vi "Median Filter.vi"(0 "Values":dbl[](array[numeric])=[5737.7244576537305, 5716.134924134484, 5694.815267577043, 5673.76167217572, 5652.9704006512275, 5632.437792319555, 5612.160261218363, 5592.1342942889905, 5572.356449612099, 5552.823354695204, 5533.531704810249, 5514.478261379612, 5495.659850408876, 5477.073360964807, 5458.7157436970465, 5440.584009402092, 5422.675227628114, 5404.98652531934, 5387.515085498669, 5370.258145987328, 5353.212998160276, 5336.376985736356, 5319.747503601926, 5303.3219966670285, 5287.097958752993, 5271.072931510506, 5255.2445033672175, 5239.610308503905, 5224.168025858348, 5208.915378156069, 5193.850130967058, 5178.970091787739, 5164.273109147386, 5149.757071738242, 5135.419907568635, 5121.259583138374, 5107.274102635845, 5093.461507155978, 5079.819873938706, 5066.347315627092, 5053.041979544701, 5039.902046991551, 5026.92573255817, 5014.111283457203, 5001.4569788720555, 4988.9611293221105, 4976.622076044022, 4964.438190388647, 4952.407873233138, 4940.529554407835, 4928.801692137438, 4917.222772496194, 50001.0, 50001.0, 50001.0, 50001.0, 50001.0, 50001.0, 50001.0, 50001.0, 50001.0, 50001.0, 50001.0, 50001.0, 50001.0, 50001.0, 50001.0, 50001.0, 50001.0, 50001.0, 50001.0, 50001.0, 50001.0, 50001.0, 50001.0, 50001.0, 50001.0, 50001.0, 50001.0, 50001.0, 50001.0, 50001.0, 50001.0, 50001.0, 50001.0, 50001.0, 50001.0, 50001.0, 50001.0, 50001.0, 50001.0, 50001.0, 50001.0, 50001.0, 50001.0, 50001.0, 50001.0, 50001.0, 50001.0, 50001.0, 50001.0, 50001.0, 50001.0, 50001.0, 50001.0, 50001.0, 50001.0, 50001.0, 50001.0, 50001.0, 50001.0, 50001.0, 50001.0, 50001.0, 50001.0, 50001.0, 50001.0, 50001.0, 50001.0, 50001.0, 50001.0, 50001.0, 50001.0, 50001.0, 50001.0, 50001.0, 50001.0, 50001.0, 50001.0, 50001.0, 50001.0, 50001.0, 50001.0, 50001.0, 50001.0, 50001.0, 50001.0, 50001.0, 50001.0, 50001.0, 50001.0, 50001.0, 50001.0, 50001.0, 4138.36385992044, 4148.764027757794, 4159.2959873554555, 4169.961147536824, 4180.760943269987, 4191.6968361984045, 4202.7703151853475, 4213.982896872684, 4225.336126254318, 4236.831577264759, 4248.470853383298, 4260.255588254225, 4272.187446323593, 4284.268123493028, 4296.499347791133, 4308.88288006296, 4321.420514678189, 4334.114080258547, 4346.965440425061, 4359.976494565826, 4373.149178624846, 4386.485465912698, 4399.987367939662, 4413.656935272053, 4427.496258412496, 4441.507468704933, 4455.69273926514, 4470.054285937593, 4484.594368279553, 4499.315290573274, 4514.219402867235, 4529.309102047392, 4544.586832939442, 4560.055089443108, 4575.716415699603, 4591.573407293312, 4607.628712488913, 4623.885033505139, 4640.345127826415, 4657.011809553725, 4673.887950796052, 4690.976483103799, 4708.280398945661, 4725.802753230531, 4743.546664875976, 4761.515318424989, 4779.711965712726, 4798.139927585015, 4816.802595670585, 4835.703434208887, 4854.845981935558, 4874.233854027718, 4893.870744111253, 4913.760426332378, 4933.906757495931, 4954.3136792729265, 4974.985220479884, 4995.925499432786, 5017.13872637844, 5038.629206006256, 5060.401340043521, 5082.459629937463, 5104.808679627467, 5127.45319841095, 5150.398003906725, 5173.648025119562, 5197.208305610149, 5221.084006774594, 5245.280411237951, 5269.802926366389, 5294.657087902874, 5319.8485637314425, 5345.3831577754045, 5371.266814035074, 5397.505620770815, 5424.105814837618, 5451.0737861775815, 5478.416082477071, 5506.13941399559, 5534.250658573846, 5549.557682605477, 5530.795421099543, 5512.264189130301, 5493.960970097327, 5475.882806682313, 5458.026799481461, 5440.39010567648, 5422.969937742926, 5405.763562194633, 5388.76829836313, 5371.981517210878, 5355.400640177337, 5339.023138056677, 5322.846529906315, 5306.868381985135, 5291.086306720595, 5275.497961703783, 5260.101048711517, 5244.89331275472, 5229.87254115221, 5215.036562629184, 5200.383246439579, 5185.910501511686, 5171.61627561618, 5157.498554556048, 5143.555361377653, 5129.784755602323, 5116.184832477928, 5102.753722249765, 5089.489589450239, 5076.390632206813, 5063.455081567598, 5050.681200844234, 5038.067284971389, 5025.61165988255, 5013.312681901523, 5001.168737149321, 4989.178240965867, 4977.3396373462, 4965.65139839078, 4954.112023769381, 4942.720040198377, 4931.474000930882, 4920.372485259511, 4909.414098031347, 4898.597469174825, 4887.921253238178, 4877.3841289391785, 4866.984798725798, 4856.721988347593, 4846.594446437441, 4836.600944103415, 4826.740274530507, 4817.011252591919, 4807.412714469748, 4797.943517284711, 4788.602538734815, 4779.388676742575, 4770.300849110739, 4761.33799318617, 4752.499065531757, 4743.783041606085, 4735.188915450776, 4726.715699385184, 4718.362423708352, 4710.128136408038, 4702.011902876599, 4694.012805633611, 4686.129944055045, 4678.362434108818, 4670.709408096625, 4663.170014401837, 4655.743417243381, 4648.428796435412, 4641.225347152678, 4634.132279701415, 4627.148819295704, 4620.27420583907, 4613.507693711313, 4606.848551560343, 4600.296062099019, 4593.849521906783, 4587.50824123604, 4581.271543823179, 4575.1387667041045, 4569.109260034198, 4563.182386912619, 4557.357523210841, 4551.634057405366, 4546.011390414479, 4540.488935438993, 4535.066117806909, 4529.74237482187, 4524.517155615389, 4519.389921002744, 4514.360143342447, 4509.42730639927, 4504.590905210715, 4499.850445956889, 4495.2054458336825, 4490.655432929259, 4486.199946103709, 4481.838534871871, 4477.570759289259, 4473.396189840984, 4469.314407333715, 4465.325002790504, 4461.427577348573, 4457.621742159845, 4453.907118294343, 4450.28333664626, 4446.750037842781, 4443.306872155521, 4439.953499414576, 4436.689588925176, 4433.5148193868445, 4430.4288788150525, 4427.431464465356, 4424.522282759926, 4421.701049216504, 4418.967488379682, 4416.32133375455, 4413.762327742603, 4411.290221579925, 4408.904775277658, 4406.605757564607, 4404.392945832097, 4402.266126080971, 4400.225092870728, 4398.269649270773, 4396.3996068137785, 4394.614785451099, 4392.915013510273, 4391.3001276545165, 4389.769972844287, 4388.324402300797, 4386.963277471562, 4385.686467997874, 4384.493851684276, 4383.385314469936, 4382.360750401986, 4381.4200616107555, 4380.563158286937, 4379.789958660625, 4379.100388982257, 4378.494383505442, 4318.089443218968, 4259.354415571307, 4202.274715166657, 4146.782541635128, 4092.81375099801, 4040.3076125210273, 3989.206584716025, 3939.456108754673, 3891.0044177352534, 3843.8023604011582, 3797.803238049603, 3752.9626534931886, 3709.2383710479176, 3666.590186619663, 3624.9798070495417, 3584.370737957352, 3544.7281793928305, 3506.018928667954, 3468.211289800222, 3431.274989048047, 3395.1810960654793, 3359.901950244804, 3325.4110918531687, 3291.6831976030867, 3258.694020327309, 3226.4203324562004, 3194.8398730209824, 3163.9312979287515, 3133.674133276207, 3104.04873148743, 3075.036230078591, 3046.6185128677234, 3018.7781734621517, 2991.4984808690338, 2964.763347086374, 2938.557296542719, 2912.865437263675, 2887.6734336524614, 2862.96748078007, 2838.734280088278, 2814.961016415716, 2791.6353362637296, 2768.745327224661, 2746.279498500686, 2724.2267624463116, 2702.576417072348, 2681.318129453483, 50001.0, 50001.0, 50001.0, 50001.0, 50001.0, 50001.0, 50001.0, 50001.0, 50001.0, 50001.0, 50001.0, 50001.0, 50001.0, 50001.0, 50001.0, 50001.0, 50001.0, 50001.0, 50001.0, 50001.0, 50001.0, 50001.0, 50001.0, 50001.0, 50001.0, 50001.0, 50001.0, 50001.0, 50001.0, 50001.0, 50001.0, 50001.0, 50001.0, 50001.0, 50001.0, 50001.0, 50001.0, 50001.0, 50001.0, 50001.0, 50001.0, 50001.0, 50001.0, 50001.0, 50001.0, 50001.0, 50001.0, 50001.0, 50001.0, 50001.0, 50001.0, 50001.0, 50001.0, 50001.0, 50001.0, 50001.0, 50001.0, 50001.0, 50001.0, 50001.0, 50001.0, 50001.0, 50001.0, 50001.0, 50001.0, 50001.0, 50001.0, 50001.0, 50001.0, 50001.0, 50001.0, 50001.0, 50001.0, 50001.0, 50001.0, 50001.0, 50001.0, 50001.0, 50001.0, 50001.0, 50001.0, 50001.0, 50001.0, 50001.0, 50001.0, 50001.0, 50001.0, 50001.0, 50001.0, 50001.0, 50001.0, 50001.0, 50001.0, 50001.0, 50001.0, 50001.0, 50001.0, 50001.0, 50001.0, 50001.0, 50001.0, 50001.0, 50001.0, 50001.0, 50001.0, 50001.0, 50001.0, 50001.0, 50001.0, 50001.0, 50001.0, 50001.0, 50001.0, 50001.0, 50001.0, 50001.0, 50001.0, 50001.0, 50001.0, 50001.0, 50001.0, 50001.0, 50001.0, 50001.0, 50001.0, 50001.0, 50001.0, 50001.0, 50001.0, 50001.0, 50001.0, 50001.0, 50001.0, 50001.0, 50001.0, 50001.0, 50001.0, 50001.0, 50001.0, 50001.0, 50001.0, 50001.0, 50001.0, 50001.0, 50001.0, 50001.0, 50001.0, 50001.0, 50001.0, 50001.0, 50001.0, 50001.0, 50001.0, 50001.0, 50001.0, 50001.0, 50001.0, 50001.0, 50001.0, 50001.0, 50001.0, 50001.0, 50001.0, 50001.0, 50001.0, 50001.0, 50001.0, 50001.0, 50001.0, 50001.0, 50001.0, 50001.0, 50001.0, 50001.0, 50001.0, 50001.0, 50001.0, 50001.0, 50001.0, 50001.0, 50001.0, 50001.0, 50001.0, 50001.0, 50001.0, 50001.0, 50001.0, 50001.0, 50001.0, 50001.0, 50001.0, 50001.0, 50001.0, 50001.0, 50001.0, 50001.0, 50001.0, 50001.0, 50001.0, 50001.0, 50001.0, 50001.0, 50001.0, 50001.0, 50001.0, 50001.0, 50001.0, 50001.0, 50001.0, 50001.0, 5839.845734528361, 5808.028417270368, 5776.665306247959, 5745.747898186631, 5715.2679068598545, 5685.21725627468, 5655.588074113117, 5626.372685418222, 5597.563606514182, 5569.153539150442, 5541.1353648603235, 5513.5021395249705, 5486.247088134002, 5459.363599734618, 5432.845222561315, 5406.685659338711, 5380.878762750365, 5355.4185310668045, 5330.299103926267, 5305.514758261971, 5281.059904370039, 5256.929082112468, 5233.116957249686, 5209.618317897682, 5186.428071104781, 5163.54123954331, 5140.952958311783, 5118.658471843292, 5096.653130916033, 5074.932389762007, 5053.491803270277, 5032.327024281081, 5011.433800967442, 4990.807974301041, 4970.445475599103, 4950.342324149441, 4930.4946249106415, 4910.8985662847435, 50001.0, 50001.0, 50001.0, 50001.0, 50001.0, 50001.0, 50001.0, 50001.0, 50001.0, 50001.0, 50001.0, 50001.0, 50001.0, 50001.0, 50001.0, 50001.0, 50001.0, 50001.0, 50001.0, 50001.0, 50001.0, 50001.0, 50001.0, 50001.0, 3500.104973160423, 3480.5640700047893, 3461.3056795485822, 3442.3244107401415, 3423.6150124568376, 3405.172369034205, 3386.9914959657904, 3369.067535766175, 3351.3957539899607, 3333.97153539993, 3316.7903802778974, 3299.847900872101, 3283.139817975284, 3266.66195762788, 3250.4102479410144, 3234.3807160342935, 3218.5694850835152, 3202.9727714738524, 3187.5868820539636, 3172.4082114870957, 3157.4332396950194, 3142.6585293911553, 3128.080723699237, 3113.6965438540915, 3099.502786981212, 3085.496323952078, 3071.674097312154, 3058.03311927878, 3044.5704698061327, 3031.2832947147617, 3018.1688038831567, 3005.2242694989304, 2992.4470243673995, 2979.834460275363, 2967.3840264079768, 2970.937817541763, 2980.912351369144, 2991.0112235651386, 3001.2360886636015, 3011.5886345895447, 3022.0705834598944, 3032.6836924078866, 3043.42975443197, 3054.310599269991, 3065.3280942995816, 3076.4841454656516, 3087.780698235946, 3099.219738585617, 3110.8032940118933, 3122.5334345798783, 3134.4122740006137, 3146.44197074253, 3158.6247291775594, 3170.9628007630813, 3183.4584852610983, 50001.0, 50001.0, 50001.0, 50001.0, 50001.0, 50001.0, 50001.0, 50001.0, 50001.0, 50001.0, 50001.0, 50001.0, 50001.0, 50001.0, 50001.0, 50001.0, 50001.0, 50001.0, 50001.0, 50001.0, 50001.0, 50001.0, 50001.0, 50001.0, 50001.0, 50001.0, 50001.0, 50001.0, 50001.0, 50001.0, 50001.0, 50001.0, 50001.0, 50001.0, 50001.0, 50001.0, 50001.0, 50001.0, 50001.0, 50001.0, 50001.0, 50001.0, 50001.0, 50001.0, 50001.0, 50001.0, 50001.0, 50001.0, 50001.0, 50001.0, 50001.0, 50001.0, 50001.0, 50001.0, 50001.0, 50001.0, 50001.0, 50001.0, 50001.0, 50001.0, 50001.0, 50001.0, 50001.0, 50001.0, 50001.0, 50001.0, 50001.0, 50001.0, 50001.0, 50001.0, 50001.0, 50001.0, 50001.0, 50001.0, 50001.0, 50001.0, 50001.0, 50001.0, 50001.0, 50001.0, 50001.0, 50001.0, 50001.0, 50001.0, 50001.0, 50001.0, 50001.0, 50001.0, 50001.0, 50001.0, 50001.0, 50001.0, 50001.0, 50001.0, 50001.0, 50001.0, 50001.0, 50001.0, 50001.0, 50001.0, 50001.0, 50001.0, 50001.0, 50001.0, 50001.0, 50001.0, 50001.0, 50001.0, 50001.0, 50001.0, 50001.0, 50001.0, 50001.0, 50001.0, 50001.0, 50001.0, 50001.0, 50001.0, 50001.0, 50001.0, 50001.0, 50001.0, 50001.0, 50001.0, 50001.0, 50001.0, 50001.0, 50001.0, 2455.5451274597576, 2357.0220066494157, 2266.1414196213445, 2182.0488805161076, 2104.0127111934958, 2031.4027439259266, 1963.673307576685, 1909.7409526396264, 1902.022359973132, 1894.401830059512, 1886.8779004739342, 1879.4491399678286, 1872.114147667534, 1864.871552297861, 1857.7200114295385, 1850.658210749831, 1843.68486335542, 1836.7987090667532, 1829.9985137632277, 1823.2830687382996, 1816.6511900739633, 1810.101718033892, 1803.6335164745988, 1797.2454722739483, 1790.936494776534, 1784.7055152552518, 1778.5514863885612, 1772.4733817529207, 1766.4701953299098, 1760.5409410274128, 1754.6846522146132, 1748.9003812701771, 1743.1871991432745, 1737.5441949269648, 1731.9704754435836, 1726.4651648417887, 1721.0274042047222, 1715.6563511691966, 1710.3511795552524, 1705.1110790060354, 1699.935254637449, 1694.8229266974606, 1689.7733302345723, 1684.7857147753496, 1679.8593440105944, 1674.9934954899713, 1670.1874603247966, 1665.4405428987382, 1660.7520605862303, 1656.121343478289, 1651.5477341155893, 1647.0305872285144, 1642.5692694840595, 1638.1631592392498, 1633.8116463010456, 1629.5141316924044, 1625.2700274243718, 1621.0787562741025, 1616.939751568437, 1612.8524569731358, 1608.8163262873668, 1604.8308232434927, 1600.8954213118373, 1597.0096035104348, 1598.765431241431, 1600.9707843753438, 1603.2127951083971, 1605.4917032157155, 1607.8077532292582, 1610.161194505086, 1612.5522812922677, 1614.9812728034733, 1617.4484332872653, 1619.9540321022057, 1622.4983437926896, 1625.0816481666675, 1627.7042303752385, 1630.3663809941645, 1633.0683961073655, 1635.8105773924349, 1638.5932322082149, 1641.4166736845048, 1644.2812208139321, 1647.1871985460343, 1650.1349378836435, 1653.124775981586, 1656.1570562477673, 1659.232128446739, 1662.350348805751], 1 "Median Window Size":i32=5) -> (2 "Filtered Values":dbl[](array[numeric]))   [LabVIEW 2017]
uses:
  <vilib>/Analysis/NI_AALBase.lvlib
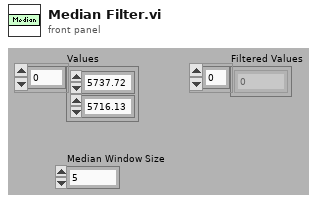
[diagram p1: front panel]
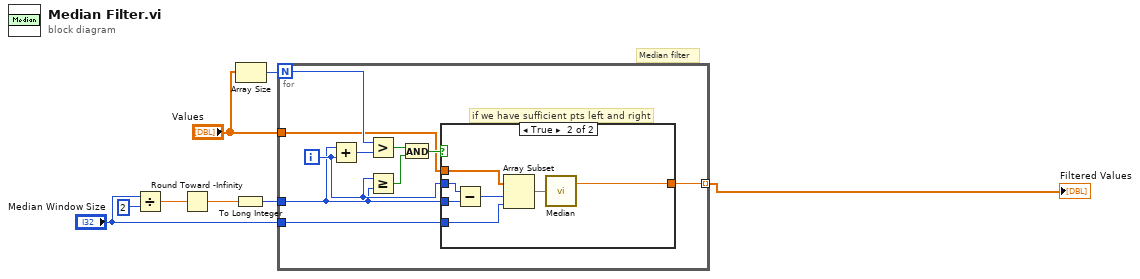
[diagram p0: block diagram]
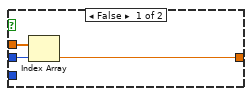
[diagram p2: hidden frame]
diagram:
  # "Median filter"
  n1 = Divide(x="Median Window Size", y=2) -> (x/y=w2:dbl)
  n2 = Round Toward -Infinity(1:w2) -> (0:w3:dbl)
  n3 = To Long Integer(number=w3) -> (32bit integer=w4:i32)
  n4 = Array Size(array="Values") -> (size(s)=w7:i32)
  n5 = for {
    N: w7 -> [w17]
    tunnel: "Values" -> [w13]
    tunnel: w4 -> [w11]
    tunnel: "Median Window Size" -> [w10]
    tunnel: [w9] -> w8 mode=indexing
    i -> [w12]
    # "if we have sufficient pts left and right"
    n6 = Add(x=w11, y=w12) -> (x+y=w18:i32)
    n7 = Greater?(x=w17, y=w18) -> (0:w15:bool)
    n8 = Greater Or Equal?(x=w12, y=w11) -> (x >= y?=w16:bool)
    n9 = And(x=w15, y=w16) -> (x .and. y?=w14:bool)
    n10 = case shown="True" w14 {
      tunnel: w13 -> [w21 w28]
      tunnel: w12 -> [w20 w27]
      tunnel: [w19 w22] -> w9
      tunnel: w11 -> [_ w26]
      tunnel: w10 -> [_ w24]
      frame False {
        n11 = Index Array(array=w21, index=w20) -> (element=w19:dbl)
      }
      frame True {
        n12 = Subtract(x=w27, y=w26) -> (x-y=w25:i32)
        n13 = Array Subset(array=w28, index=w25, length=w24) -> (w23:dbl[])
        n14 = call <vilib>:"Median.vi"("X"=w23) -> ("median"=w22:dbl)  [unwired: 1 out]
      }
    }
  }
  "Filtered Values" <- w8
